vi "E11_Maquina de estados.vi"() -> ()   [LabVIEW 2026]
panel:
  out "String":string
  in  "stop":bool
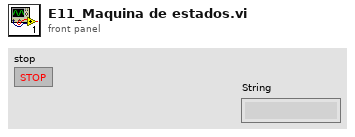
[diagram p1: front panel]
types:
  T1 = enum16{"Inicio", "Paso 1", "Paso 2", "Paso 3", "Fin"}
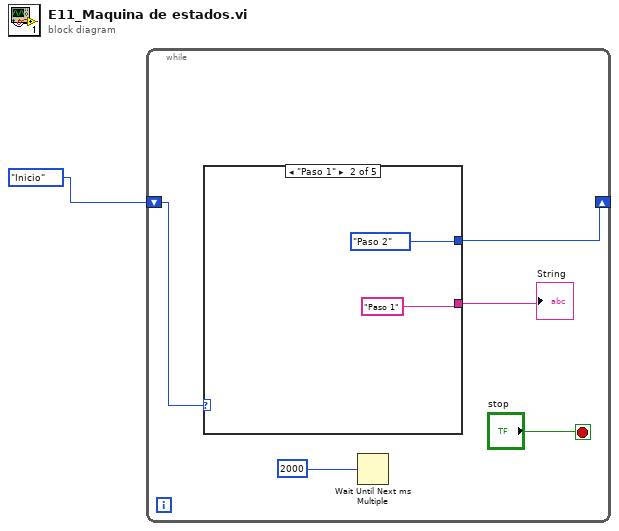
[diagram p0: block diagram]
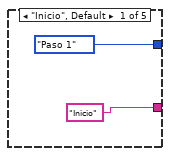
[diagram p2: hidden frame]
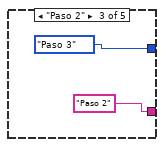
[diagram p3: hidden frame]
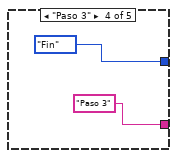
[diagram p4: hidden frame]
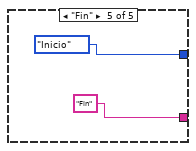
[diagram p5: hidden frame]
diagram:
  n1 = while {
    shift-right: [w4] -> _
    shift-left: T1."Inicio" -> [w5]
    stop <- "stop" stop-if-true
    n2 = case shown="\"Paso 1\"" w5 {
      tunnel: [T1."Paso 1" T1."Paso 2" T1."Paso 3" T1."Fin" T1."Inicio"] -> w4
      tunnel: ["Inicio" "Paso 1" "Paso 2" "Paso 3" "Fin"] -> w3
      frame "Inicio", Default {
      }
      frame "Paso 1" {
      }
      frame "Paso 2" {
      }
      frame "Paso 3" {
      }
      frame "Fin" {
      }
    }
    "String" <- w3
    n3 = Wait Until Next ms Multiple(millisecond multiple=2000) -> ()  [unwired: 1 out]
  }
